vi "Read File ini.vi"(8 "error in (no error)":errorcluster, 11 "Telegram Class in":refnum<class "Telegram Class.lvclass">) -> (0 "error out":errorcluster, 3 "Telegram Class out":refnum<class "Telegram Class.lvclass">)   [LabVIEW 2015, in "Telegram Library.lvlib" / "Telegram Class.lvclass"]
doc: "Created IvanLis by LabVIEW Portal\nProfile: http://labviewportal.org/memberlist.php?mode=viewprofile&u=987\neMail: IvanLisanov@gMail.com\nTelegram: https://t.me/IvanLis"
uses:
  Telegram Class.lvclass
  Telegram Class.lvclass/Telegram Class.ctl
  <vilib>/Utility/config.llb/Read Key (String).vi
  <vilib>/Utility/config.llb/Read Key (Boolean).vi
  <vilib>/Utility/config.llb/Read Key (I32).vi
  <vilib>/Utility/config.llb/NI_LVConfig.lvlib
  Telegram Library.lvlib
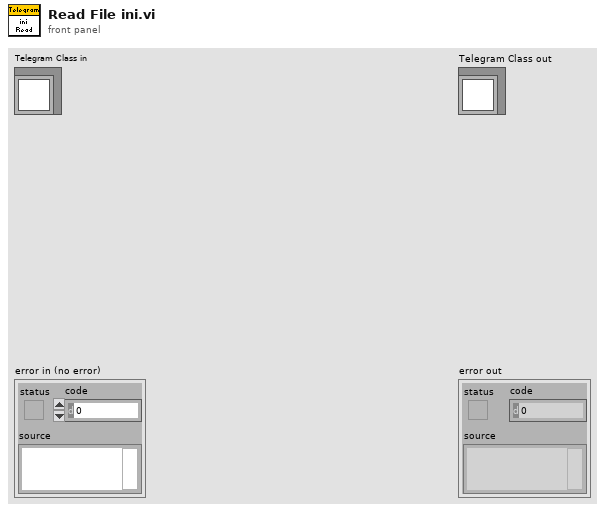
[diagram p1: front panel]
types:
  T1 = typedef "NI_LVConfig.lvlib/Config Data RefNum.ctl" = refnum<k1>
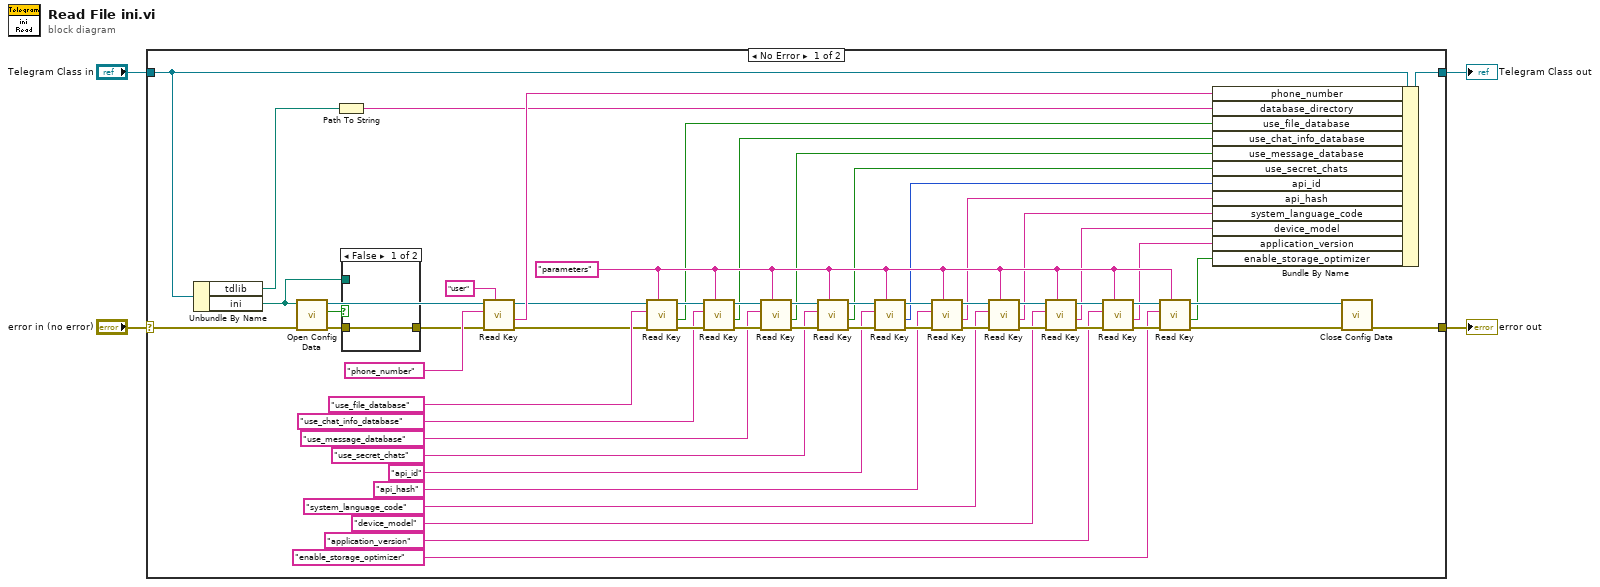
[diagram p0: block diagram]
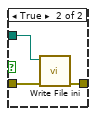
[diagram p2: hidden frame]
diagram:
  n1 = case shown="No Error" "error in (no error)" {
    selector: "error in (no error)" -> [w61 w67]
    tunnel: [w60 w67] -> w3
    tunnel: [w58 w66] -> w1
    tunnel: "Telegram Class in" -> [w59 w66]
    frame No Error {
      w31 = "parameters"
      n2 = Unbundle By Name(w59) -> ("tdlib"=w20:path, "ini"=w55:path)
      n3 = call <vilib>:"Open Config Data.vi"("error in (no error)"=w61, "configuration file path"=w55) -> ("error out"=w56:errorcluster, "file created?"=w57:bool, "refnum"=w51:T1)  [unwired: 7 in]
      n4 = Path To String(path=w20) -> (string=w7:string)
      n5 = case shown="False" w57 {
        tunnel: w56 -> [w62 w65]
        tunnel: [w62 w64] -> w52
        tunnel: w55 -> [_ w63]
        frame False {
        }
        frame True {
          n6 = call "Write File ini.vi"("error in (no error)"=w65, "ini Path"=w63) -> ("error out"=w64:errorcluster)  [unwired: 9 in]
        }
      }
      n7 = call-poly <vilib>:"Read Key.vi"("section"="user", "error in (no error)"=w52, "key"="phone_number", "refnum"=w51) -> ("error out"=w5:errorcluster, "value"=w50:string, "refnum out"=w6:T1)  [unwired: 4 in, 1 out]
      n8 = call-poly <vilib>:"Read Key.vi"("section"=w31, "error in (no error)"=w5, "key"="use_file_database", "refnum"=w6) -> ("error out"=w36:errorcluster, "value"=w8:bool, "refnum out"=w47:T1)  [unwired: 4 in, 1 out]
      n9 = call-poly <vilib>:"Read Key.vi"("section"=w31, "error in (no error)"=w36, "key"="use_chat_info_database", "refnum"=w47) -> ("error out"=w35:errorcluster, "value"=w9:bool, "refnum out"=w46:T1)  [unwired: 4 in, 1 out]
      n10 = call-poly <vilib>:"Read Key.vi"("section"=w31, "error in (no error)"=w35, "key"="use_message_database", "refnum"=w46) -> ("error out"=w34:errorcluster, "value"=w10:bool, "refnum out"=w45:T1)  [unwired: 4 in, 1 out]
      n11 = call-poly <vilib>:"Read Key.vi"("section"=w31, "error in (no error)"=w34, "key"="use_secret_chats", "refnum"=w45) -> ("error out"=w33:errorcluster, "value"=w11:bool, "refnum out"=w44:T1)  [unwired: 4 in, 1 out]
      n12 = call-poly <vilib>:"Read Key.vi"("section"=w31, "error in (no error)"=w33, "key"="api_id", "refnum"=w44) -> ("error out"=w32:errorcluster, "value"=w12:i32, "refnum out"=w43:T1)  [unwired: 4 in, 1 out]
      n13 = call-poly <vilib>:"Read Key.vi"("section"=w31, "error in (no error)"=w32, "key"="api_hash", "refnum"=w43) -> ("error out"=w49:errorcluster, "value"=w13:string, "refnum out"=w48:T1)  [unwired: 4 in, 1 out]
      n14 = call-poly <vilib>:"Read Key.vi"("section"=w31, "error in (no error)"=w49, "key"="system_language_code", "refnum"=w48) -> ("error out"=w39:errorcluster, "value"=w14:string, "refnum out"=w42:T1)  [unwired: 4 in, 1 out]
      n15 = call-poly <vilib>:"Read Key.vi"("section"=w31, "error in (no error)"=w39, "key"="device_model", "refnum"=w42) -> ("error out"=w38:errorcluster, "value"=w15:string, "refnum out"=w41:T1)  [unwired: 4 in, 1 out]
      n16 = call-poly <vilib>:"Read Key.vi"("section"=w31, "error in (no error)"=w38, "key"="application_version", "refnum"=w41) -> ("error out"=w37:errorcluster, "value"=w16:string, "refnum out"=w40:T1)  [unwired: 4 in, 1 out]
      n17 = call-poly <vilib>:"Read Key.vi"("section"=w31, "error in (no error)"=w37, "key"="enable_storage_optimizer", "refnum"=w40) -> ("error out"=w18:errorcluster, "value"=w17:bool, "refnum out"=w19:T1)  [unwired: 4 in, 1 out]
      n18 = Bundle By Name(cluster=w59, "phone_number"=w50, "database_directory"=w7, "use_file_database"=w8, "use_chat_info_database"=w9, "use_message_database"=w10, "use_secret_chats"=w11, "api_id"=w12, "api_hash"=w13, "system_language_code"=w14, "device_model"=w15, "application_version"=w16, "enable_storage_optimizer"=w17) -> (w58:refnum<class "Telegram Class.lvclass">)
      n19 = call <vilib>:"Close Config Data.vi"("error in (no error)"=w18, "refnum"=w19) -> ("error out"=w60:errorcluster)  [unwired: 8 in, 1 out]
    }
    frame Error {
    }
  }
  "error out" <- w3
  "Telegram Class out" <- w1
